vi "RobotLiftOutput.vi"   [LabVIEW 2017, in "RobotLift.lvclass"]
uses:
  Subsystem/RobotLift/RobotLift.lvclass
  SubsystemData/RobotLiftData/RobotLiftData.lvclass
  R:/Documents/github/FRC4080/2018-robot-main/SubsystemData/SubsystemData.lvclass
  <vilib>/Rock Robotics/WPI/Solenoid/WPI_SolenoidValue.ctl
  <vilib>/Rock Robotics/WPI/ThirdParty/Phoenix-LabVIEW/Motor Controller/Controls/CTRE_Phoenix_MotorControl_ControlMode.ctl
  <vilib>/Rock Robotics/WPI/Solenoid/WPI_SolenoidSetEnum.vi
types:
  T1 = typedef "WPI_SolenoidValue.ctl" = enum16{"Off", "On", "Forward", "Reverse"}
  T2 = typedef "CTRE_Phoenix_MotorControl_ControlMode.ctl" = u16
  T3 = typedef "RobotLiftData.lvclass/RobotLiftOutput.ctl" = cluster{"LeftRobotLiftSetting":dbl, "RightRobotLiftSetting":dbl, "RampReleaseSetting":bool}
  T4 = typedef "WPI_SolenoidDevRef.ctl" = cluster{"DevStatus":errorcluster, "Pneumatics Control Module":u8, "Forward Solenoid Channel":T5, "Reverse Solenoid Channel":T5}
  T5 = typedef "WPI_SolenoidChannel.ctl" = enum8{"Solenoid 0", "Solenoid 1", "Solenoid 2", "Solenoid 3", "Solenoid 4", "Solenoid 5", "Solenoid 6", "Solenoid 7", "Invalid"}
  T6 = typedef "WPI_MotorControlDeviceRef.ctl" = cluster{"DeviceStatus":errorcluster, "Type":T7, "PWM":cluster{"PWM Channel":T8, "DeadBand":T9}, "CAN":cluster{"Device Number":u8, "SetOutput VI Ref":variant, "GetOutput VI Ref":variant, "Enable VI Ref":variant, "Disable VI Ref":variant, "Data":variant}, "Invert":bool, "DIO PWM":cluster{"PWM \"Enable\" Channel":T8, "DIOChannel":T10, "PWM Rate":dbl}}
  T7 = typedef "WPI_MotorControlType.ctl" = enum16{"PWM", "CAN", "DIO PWM"}
  T8 = typedef "FPGA_DIOPWMChannel.ctl" = enum8{"PWM 0", "PWM 1", "PWM 2", "PWM 3", "PWM 4", "PWM 5", "PWM 6", "PWM 7", "PWM 8", "PWM 9", "PWM MXP 0", "PWM MXP 1", "PWM MXP 2", "PWM MXP 3", "PWM MXP 4", "PWM MXP 5", "PWM MXP 6", "PWM MXP 7", "PWM MXP 8", "PWM MXP 9", "Invalid"}
  T9 = typedef "WPI_PWMDeadband.ctl" = cluster{"Name":string, "maxPositivePwm":i32, "minPositivePwm":i32, "centerPwm":i32, "maxNegativePwm":i32, "minNegativePwm":i32, "angularRange":u16}
  T10 = typedef "FPGA_DIOChannel.ctl" = enum8{"DIO 0", "DIO 1", "DIO 2", "DIO 3", "DIO 4", "DIO 5", "DIO 6", "DIO 7", "DIO 8", "DIO 9", "DIO MXP 0", "DIO MXP 1", "DIO MXP 2", "DIO MXP 3", "DIO MXP 4", "DIO MXP 5", "DIO MXP 6", "DIO MXP 7", "DIO MXP 8", "DIO MXP 9", "DIO MXP 10", "DIO MXP 11", "DIO MXP 12", "DIO MXP 13", "DIO MXP 14", "DIO MXP 15", "SPI Port CS1", "SPI Port CS2", "SPI Port CS3", "SPI Port MISO", "SPI Port MOSI", "Invalid"}
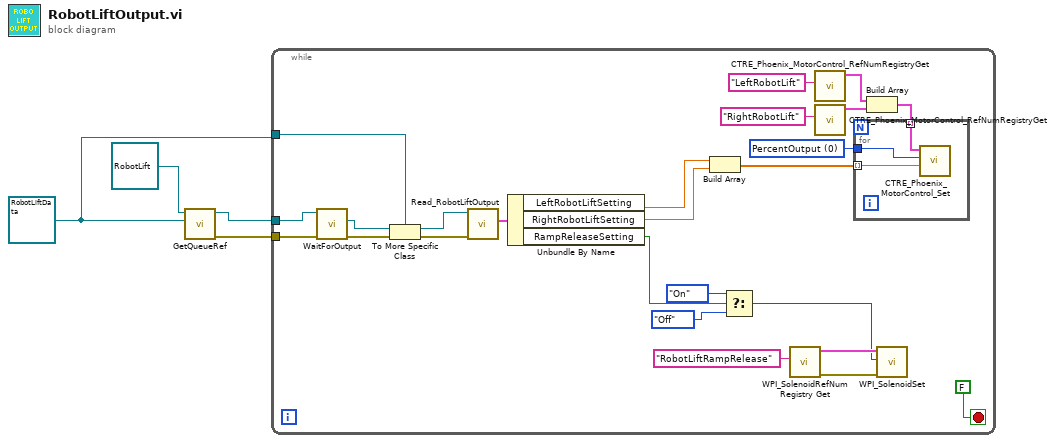
[diagram p0: block diagram]
diagram:
  w1 = refnum<class "RobotLiftData.lvclass"> refnum ("RobotLiftData.lvclass")
  n1 = call-dynamic "GetQueueRef.vi"("SubsystemData.lvclass"=w1, "Subsystem in"=refnum<class "RobotLift.lvclass"> refnum ("RobotLift.lvclass")) -> ("error out"=w3:errorcluster, "Subsystem out"=w2:refnum<class "RobotLift.lvclass">)  [unwired: 8 in]
  n2 = while {
    tunnel: w3 -> [w7]
    tunnel: w2 -> [w8]
    tunnel: w1 -> [w12]
    stop <- FALSE stop-if-true
    w26 = T2 0 items=["PercentOutput"=0, "Position"=1, "Velocity"=2, "Current"=3, "Follower"=5, "MotionProfile"=6, "MotionMagic"=7, "MotionMagicArc"=8, "MotionProfileArc"=10, "Disabled"=15] ("Control Mode")
    n3 = call-dynamic "WaitForOutput.vi"("error in (no error)"=w7, "Subsystem in"=w8) -> ("error out"=w6:errorcluster, "Subsystem Output"=w5:refnum<class "SubsystemData.lvclass">)  [unwired: 7 in, 1 out]
    n4 = To More Specific Class(target class=w12, reference=w5, error in=w6) -> (specific class reference=w11:refnum<class "RobotLiftData.lvclass">, error out=w10:errorcluster)
    n5 = call-dynamic "Read_RobotLiftOutput.vi"("error in (no error)"=w10, "RobotLiftData in"=w11) -> ("RobotLiftOutput"=w9:T3)  [unwired: 7 in, 2 out]
    n6 = Unbundle By Name(w9) -> ("LeftRobotLiftSetting"=w17:dbl, "RightRobotLiftSetting"=w18:dbl, "RampReleaseSetting"=w16:bool)
    n7 = Build Array(w17, w18) -> (w22:dbl[])
    n8 = Select(t=WPI_SolenoidValue."On", s=w16, f=WPI_SolenoidValue."Off" ("Value")) -> (s? t:f=w14:T1)
    n9 = call <vilib>:"WPI_SolenoidRefNum Registry Get.vi"("refnum name"="RobotLiftRampRelease") -> ("error out"=w27:errorcluster, "SolenoidDevRef"=w28:T4)  [unwired: 9 in]
    n10 = call <vilib>:"CTRE_Phoenix_MotorControl_RefNumRegistryGet.vi"("refnum name"="LeftRobotLift") -> ("PhoenixMotorControlDevRef"=w25:T6)  [unwired: 9 in, 1 out]
    n11 = call <vilib>:"CTRE_Phoenix_MotorControl_RefNumRegistryGet.vi"("refnum name"="RightRobotLift") -> ("PhoenixMotorControlDevRef"=w24:T6)  [unwired: 9 in, 1 out]
    n12 = Build Array(w25, w24) -> (w23:T6[])
    n13 = for {
      tunnel: w26 -> [w32]
      tunnel: w23 -> [w31] mode=indexing
      tunnel: w22 -> [w30] mode=indexing
      n14 = call <vilib>:"CTRE_Phoenix_MotorControl_Set.vi"("Output"=w30, "Control Mode"=w32, "PhoenixMotorControlDevRef"=w31) -> ()  [unwired: 7 in, 2 out]
    }
    n15 = call-poly <vilib>:"WPI_SolenoidSet.vi"("error in (no error)"=w27, "Value"=w14, "SolenoidDevRef"=w28) -> ()  [unwired: 7 in, 2 out]
  }
